vi "Thev-Compute.vi"(0 "folder":path, 7 "Options":T2={"Fmin"=500.0, "Fmax"=10000.0}, 9 "probe tube path":path, 11 "error in (no error)":errorcluster) -> (4 "log":string, 8 "Result":T1, 15 "error out":errorcluster)   [LabVIEW 2015]
uses:
  Typedefs/Thev-Optimization Parameters.ctl
  Typedefs/Thev-Optimization Result.ctl
  Utility VIs/Math VIs/Z to dB, degrees (1D).vi
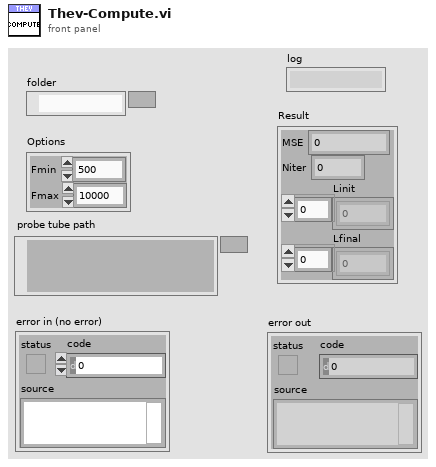
[diagram p1: front panel]
types:
  T1 = typedef "Thev-Optimization Result.ctl" = cluster{"MSE":dbl, "Niter":i32, "Linit":dbl[], "Lfinal":dbl[]}
  T2 = typedef "Thev-Optimization Parameters.ctl" = cluster{"Fmin":dbl, "Fmax":dbl}
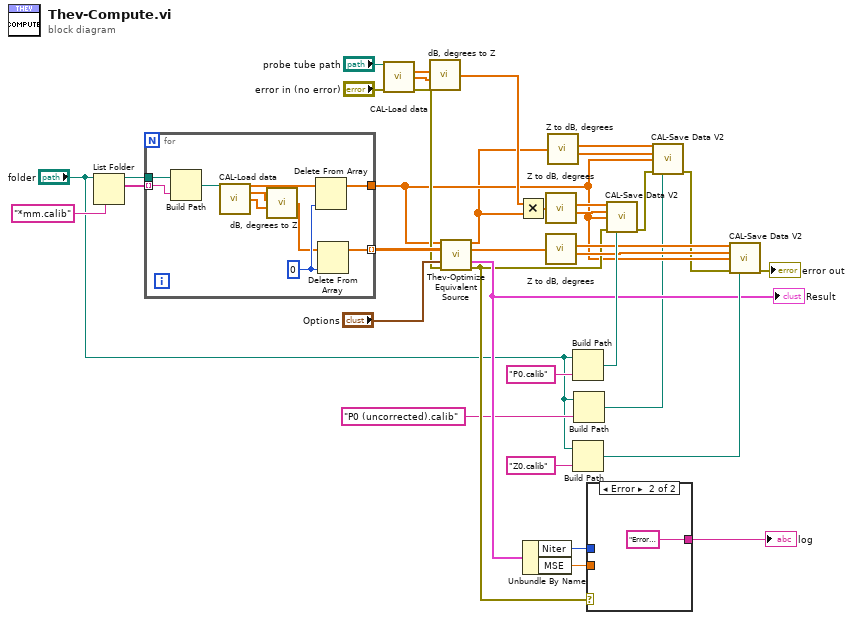
[diagram p0: block diagram]
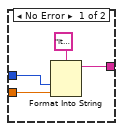
[diagram p2: hidden frame]
diagram:
  n1 = List Folder(path="folder", pattern="*mm.calib") -> (path out=w25:path, filenames=w27:string[])  [unwired: 2 in, 2 out]
  n2 = for {
    tunnel: w25 -> [w46]
    tunnel: [w39] -> w28 mode=indexing
    tunnel: [w40] -> w9
    tunnel: w27 -> [w42] mode=indexing
    w38 = 0 ("index")
    n3 = Build Path(base path=w46, name or relative path=w42) -> (appended path=w45:path)
    n4 = call "CAL-Load data.vi"("user path"=w45) -> ("Frequency (Hz)"=w41:dbl[], "Mag"=w44:dbl[], "Phase"=w43:dbl[])  [unwired: 7 in, 5 out]
    n5 = call "dB, degrees to Z.vi"("Magnitude (dB)"=w44, "Phase (degrees)"=w43) -> ("Z"=w37:cdb[])  [unwired: 5 in]
    n6 = Delete From Array(array=w41, index=w38) -> (array with subset deleted=w40:dbl[])  [unwired: 1 in, 1 out]
    n7 = Delete From Array(array=w37, index=w38) -> (array with subset deleted=w39:cdb[])  [unwired: 1 in, 1 out]
  }
  n8 = call "CAL-Load data.vi"("user path"="probe tube path", "error in (no error)"="error in (no error)") -> ("Mag"=w30:dbl[], "Phase"=w31:dbl[], "error out"=w18:errorcluster)  [unwired: 6 in, 5 out]
  n9 = call "dB, degrees to Z.vi"("Magnitude (dB)"=w30, "Phase (degrees)"=w31) -> ("Z"=w19:cdb[])  [unwired: 5 in]
  n10 = call "Thev-Optimize Equivalent Source.vi"("Frequency (Hz)"=w9, "Px"=w28, "Options"="Options", "error in (no error)"=w18) -> ("Ps"=w3:cdb[], "Zs"=w23:cdb[], "Result"=w15:T1, "error out"=w14:errorcluster)  [unwired: 8 in]
  "Result" <- w15
  n11 = Multiply(x=w19, y=w3) -> (x*y=w20:cdb[])
  n12 = Unbundle By Name(w15) -> ("Niter"=w12:i32, "MSE"=w11:dbl)
  n13 = call-poly "Z to dB, degrees.vi"("Z"=w20) -> ("Magnitude (dB)"=w24:dbl[], "Phase (degrees)"=w10:dbl[])  [unwired: 5 in]
  n14 = call-poly "Z to dB, degrees.vi"("Z"=w23) -> ("Magnitude (dB)"=w22:dbl[], "Phase (degrees)"=w21:dbl[])  [unwired: 5 in]
  n15 = call-poly "Z to dB, degrees.vi"("Z"=w3) -> ("Magnitude (dB)"=w2:dbl[], "Phase (degrees)"=w1:dbl[])  [unwired: 5 in]
  n16 = Build Path(base path="folder", name or relative path="P0.calib") -> (appended path=w35:path)
  n17 = Build Path(base path="folder", name or relative path="Z0.calib") -> (appended path=w33:path)
  n18 = Build Path(base path="folder", name or relative path="P0 (uncorrected).calib") -> (appended path=w4:path)
  n19 = case shown="Error" w14 {
    tunnel: [w47 "Error optimizing equivalent source.\n"] -> w13
    tunnel: w12 -> [w49 _]
    tunnel: w11 -> [w48 _]
    frame No Error {
      n20 = Format Into String(format string="Iterations: %d\nMSE: %.2e\nFinished.\n", w49, w48) -> (resulting string=w47:string)  [unwired: 2 in, 1 out]
    }
    frame Error {
    }
  }
  "log" <- w13
  n21 = call "CAL-Save Data V2.vi"("Mag"=w24, "Phase"=w10, "Frequency"=w9, "error in (no error)"=w14, "path"=w35) -> ("error out"=w8:errorcluster)  [unwired: 9 in, 1 out]
  n22 = call "CAL-Save Data V2.vi"("Mag"=w2, "Phase"=w1, "Frequency"=w9, "error in (no error)"=w8, "path"=w4) -> ("error out"=w7:errorcluster)  [unwired: 9 in, 1 out]
  n23 = call "CAL-Save Data V2.vi"("Mag"=w22, "Phase"=w21, "Frequency"=w9, "error in (no error)"=w7, "path"=w33) -> ("error out"=→"error out":errorcluster)  [unwired: 9 in, 1 out]
